vi "Configure Scale Offset.vi"(7 "Enable Scale Offset (Disable)":bool, 8 "error in (no error)":errorcluster, 9 "Offset (0)":dbl format="%#_7g", 10 "Scale (1)":dbl=1.0 format="%#_7g", 11 "VISA resource name":refnum<visa-resource-name>) -> (0 "error out":errorcluster, 3 "VISA resource name out":refnum<visa-resource-name>)   [LabVIEW 2013, in "Counter.lvlib" / "PICOTEST U62XXA series.lvlib"]
doc: "Configures the parameters required for performing post acquisition Scale and Offset operation.\n\n<B>Note:</B>\n\nTotalize and Volt Peak Measurements <B>does not</B> support post acquisiton Scale Offset operation."
uses:
  PICOTEST U62XXA series.lvlib
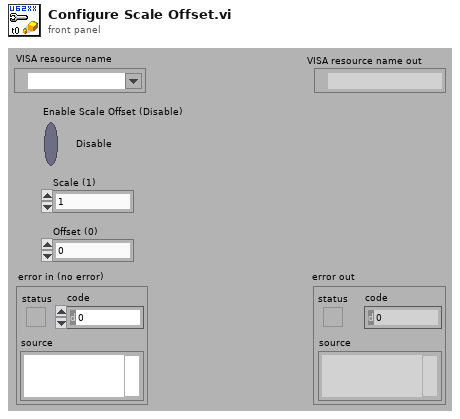
[diagram p1: front panel]
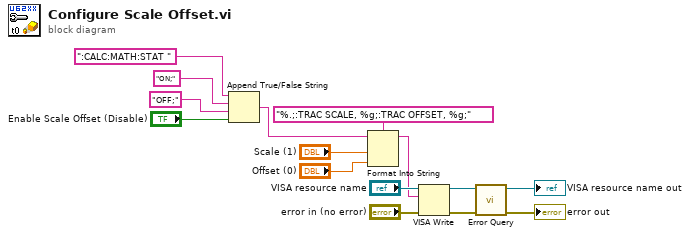
[diagram p0: block diagram]
diagram:
  n1 = Append True/False String(1:"Enable Scale Offset (Disable)", 2:"OFF;" ("false string"), 3:"ON;" ("true string"), 4:":CALC:MATH:STAT " ("string (\"\")")) -> (0:w6:string)
  n2 = Format Into String(format string="%.;:TRAC SCALE, %g;:TRAC OFFSET, %g;", initial string=w6, "Scale (1)", "Offset (0)") -> (resulting string=w5:string)  [unwired: 1 in, 1 out]
  n3 = VISA Write(VISA resource name="VISA resource name", write buffer=w5, error in (no error)="error in (no error)") -> (VISA resource name out=w4:refnum<visa-resource-name>, error out=w3:errorcluster)  [unwired: 1 out]
  n4 = call "Error Query.vi"("error in (no error)"=w3, "VISA resource name"=w4) -> ("error out"=→"error out":errorcluster, "VISA resource name out"=→"VISA resource name out":refnum<visa-resource-name>)  [unwired: 6 in, 2 out]
